vi "AlliGator Convert Calibration Map v1 to v2.vi"(8 "error in (no error)":errorcluster, 11 "Phasor Calibration Map v1":T1 {"ROI Descriptors"."Contours"."Type" items=["No Selection", "Point", "Line", "Rectangle", "Oval", "Polygon", "Freehand Region", "Annulus", "Unused2", "Unused3", "Broken Line", "Freehand Line", "Rotated Rectangle"]}) -> (0 "error out":errorcluster, 3 "Phasor Calibration Map v2":T3={"Phasor Frequency"=80000000.0, "Calibration Lifetime"=1e-09, "ROI Centers"=[], "ROI Descriptors"=[], "Map Resolution X"=0, "Map Resolution Y"=0, "z Array"=[]} {"ROI Descriptors"."Contours"."Type" items=["No Selection", "Point", "Line", "Rectangle", "Oval", "Polygon", "Freehand Region", "Annulus", "Unused2", "Unused3", "Broken Line", "Freehand Line", "Rotated Rectangle"]})   [LabVIEW 2021, in "AlliGator Phasor Calibration.lvlib"]
doc: "Phasor calibration map version conversion."
uses:
  AlliGator Phasor Calibration.lvlib
  Phasor/Phasor Calibration Map v2.ctl
  AlliGator Phasor Calibration Map v1.ctl
  Phasor/Phasor.lvlib
panel:
  # "see the AlliGator License on the block diagram (Ctrl+E or Window:Show Block Diagram)"
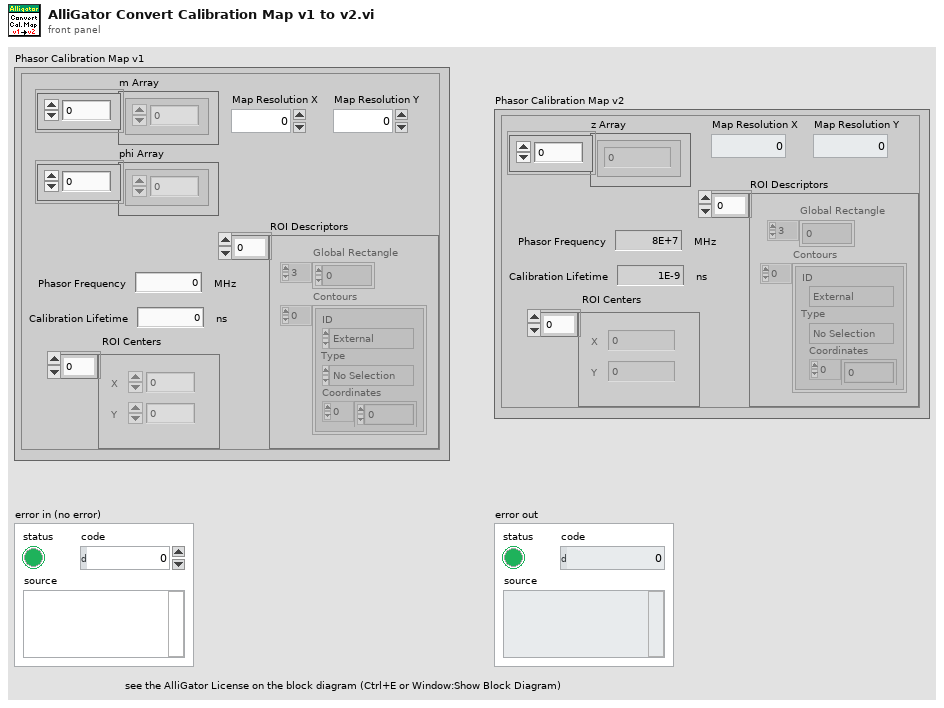
[diagram p1: front panel]
types:
  T1 = typedef "AlliGator Phasor Calibration.lvlib/AlliGator Phasor Calibration Map v1.ctl" = cluster{"m Array":dbl[], "phi Array":dbl[], "Phasor Frequency":dbl[unit], "Calibration Lifetime":dbl[unit], "ROI Centers":cluster{"X":i32, "Y":i32}[], "ROI Descriptors":T2[], "Map Resolution X":i32, "Map Resolution Y":i32}
  T2 = typedef "ROI Descriptor" = cluster{"Global Rectangle":i32[], "Contours":cluster{"ID":enum32{"External", "Internal"}, "Type":u32, "Coordinates":i32[]}[]}
  T3 = typedef "Phasor.lvlib/Phasor Calibration Map v2.ctl" = cluster{"Phasor Frequency":dbl[unit], "Calibration Lifetime":dbl[unit], "ROI Centers":cluster{"X":i32, "Y":i32}[], "ROI Descriptors":T2[], "Map Resolution X":i32, "Map Resolution Y":i32, "z Array":cdb[]}
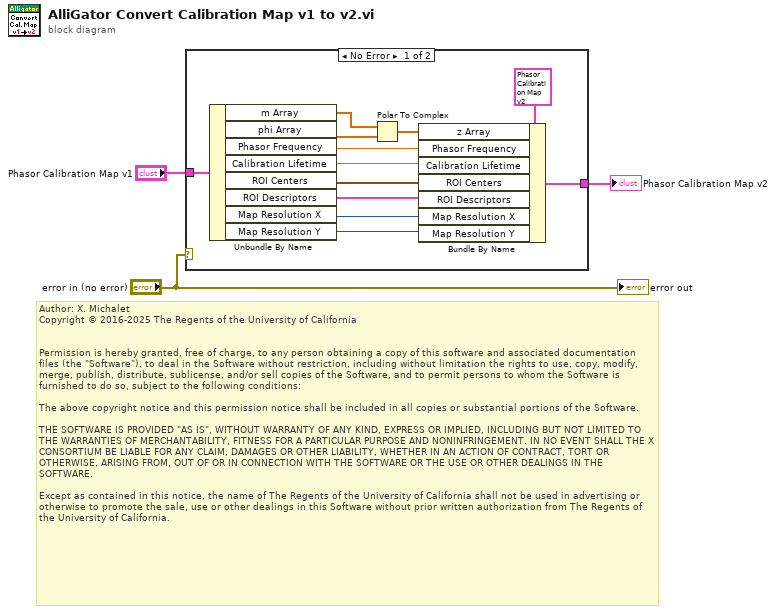
[diagram p0: block diagram]
diagram:
  # "Author: X. Michalet\nCopyright © 2016-2025 The Regents of the University of California\n \n\nPermission is hereby granted, free of charge, to any person obtaining a copy of this software and associated documentation files (the \"Software\"), to deal in the Software without restriction, including without limitation the rights to use, copy, modify, merge, publish, distribute, sublicense, and/or sell copies of the Software, and to permit persons to whom the Software is furnished to do so, subject to the following conditions:\n\nThe above copyright notice and this permission notice shall be included in all copies or substantial portions of the Software.\n\nTHE SOFTWARE IS PROVIDED \"AS IS\", WITHOUT WARRANTY OF ANY KIND, EXPRESS OR IMPLIED, INCLUDING BUT NOT LIMITED TO THE WARRANTIES OF MERCHANTABILITY, FITNESS FOR A PARTICULAR PURPOSE AND NONINFRINGEMENT. IN NO EVENT SHALL THE X CONSORTIUM BE LIABLE FOR ANY CLAIM, DAMAGES OR OTHER LIABILITY, WHETHER IN AN ACTION OF CONTRACT, TORT OR OTHERWISE, ARISING FROM, OUT OF OR IN CONNECTION WITH THE SOFTWARE OR THE USE OR OTHER DEALINGS IN THE SOFTWARE.\n\nExcept as contained in this notice, the name of The Regents of the University of California shall not be used in advertising or otherwise to promote the sale, use or other dealings in this Software without prior written authorization from The Regents of the University of California."
  n1 = case shown="No Error" "error in (no error)" {
    tunnel: "Phasor Calibration Map v1" -> [w15 _]
    tunnel: [w13 _] -> w2
    frame No Error {
      n2 = Unbundle By Name(w15) -> ("m Array"=w12:dbl[], "phi Array"=w11:dbl[], "Phasor Frequency"=w4:dbl[unit], "Calibration Lifetime"=w5:dbl[unit], "ROI Centers"=w6:cluster{"X":i32, "Y":i32}[], "ROI Descriptors"=w7:T2[], "Map Resolution X"=w8:i32, "Map Resolution Y"=w9:i32)
      n3 = Polar To Complex(1:w11, 2:w12) -> (0:w10:cdb[])
      n4 = Bundle By Name(cluster=T3 {"Phasor Frequency"=80000000.0, "Calibration Lifetime"=1e-09, "ROI Centers"=[], "ROI Descriptors"=[], "Map Resolution X"=0, "Map Resolution Y"=0, "z Array"=[]} ("Phasor Calibration Map"), "z Array"=w10, "Phasor Frequency"=w4, "Calibration Lifetime"=w5, "ROI Centers"=w6, "ROI Descriptors"=w7, "Map Resolution X"=w8, "Map Resolution Y"=w9) -> (w13:T3)
    }
    frame Error {
    }
  }
  "Phasor Calibration Map v2" <- w2
  "error out" <- "error in (no error)"
